vi "Histerisis.vi"() -> ()   [LabVIEW 2020]
panel:
  in  "x":dbl
  in  "MAX":dbl
  in  "MIN":dbl
  out "Histerísis":bool
  out "Boolean":bool
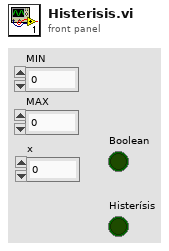
[diagram p1: front panel]
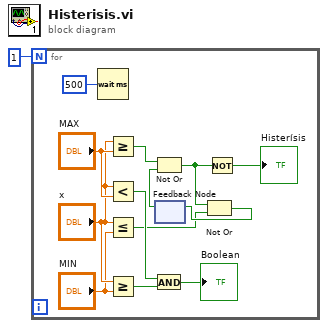
[diagram p0: block diagram]
diagram:
  n1 = for {
    N: 1 -> [_]
    n2 = Wait (ms)(milliseconds to wait=u32 500) -> ()  [unwired: 1 out]
    n3 = Greater Or Equal?(x="x", y="MAX") -> (x >= y?=w7:bool)
    n4 = Less?(x="x", y="MAX") -> (x < y?=w13:bool)
    n5 = Less Or Equal?(x="x", y="MIN") -> (x <= y?=w4:bool)
    n6 = Greater Or Equal?(x="x", y="MIN") -> (x >= y?=w10:bool)
    n7 = And(x=w13, y=w10) -> (x .and. y?=→"Boolean":bool)
    n8 = feedback #1() -> (w5:bool)  [unwired: 1 in]
    n9 = Not Or(1:w5, 2:w7) -> (0:w2:bool)
    n10 = Not Or(1:w4, 2:w2) -> (0:w6:bool)
    n11 = feedback-in #1(w6) -> ()
    n12 = Not(x=w2) -> (.not. x?=→"Histerísis":bool)
  }
